vi "Newmark-Home.vi"(0 "Table VRN IN":refnum<visa-resource-name>="COM9", 1 "Comm Active":refnum<vi>, 2 "Exceptions":refnum<vi>, 5 "StageTAGs":string[](array[string]), 7 "Velocities":cluster{"Slow":dbl, "Fast":dbl, "Accel":dbl}={"Slow"=10.0, "Fast"=25000.0, "Accel"=25000.0}, 9 "HomeReverse?":bool[](array[boolean]), 11 "Error IN":errorcluster, 12 "Quit Orgine":refnum<vi>, 13 "EndValues":i32[](array[numeric])) -> (4 "Table VRN OUT":refnum<visa-resource-name>="COM9", 15 "Error OUT":errorcluster)   [LabVIEW 2011]
panel:
  out "NumOT":i32
  out "T Home":dbl
  out "Z Home":dbl
  out "Y Home":dbl
  out "X Home":dbl
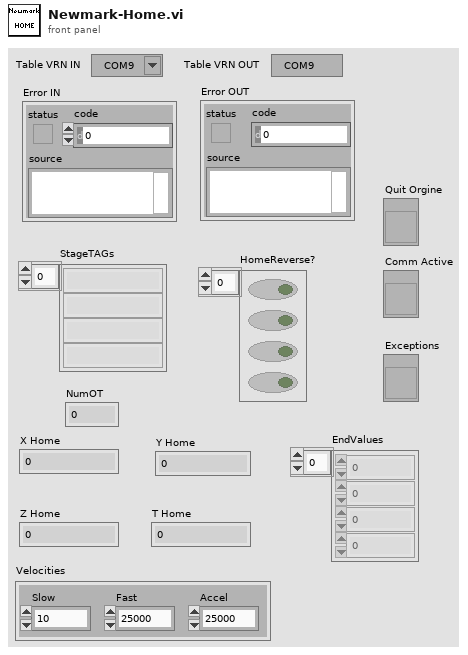
[diagram p1: front panel]
types:
  T1 = cluster{"Command Error":bool, "Slip/Stall":bool, "Overtravel":bool, "Done":bool, "nError":u32, "nSlip":u32, "nOT":u32, "nDone":u32}
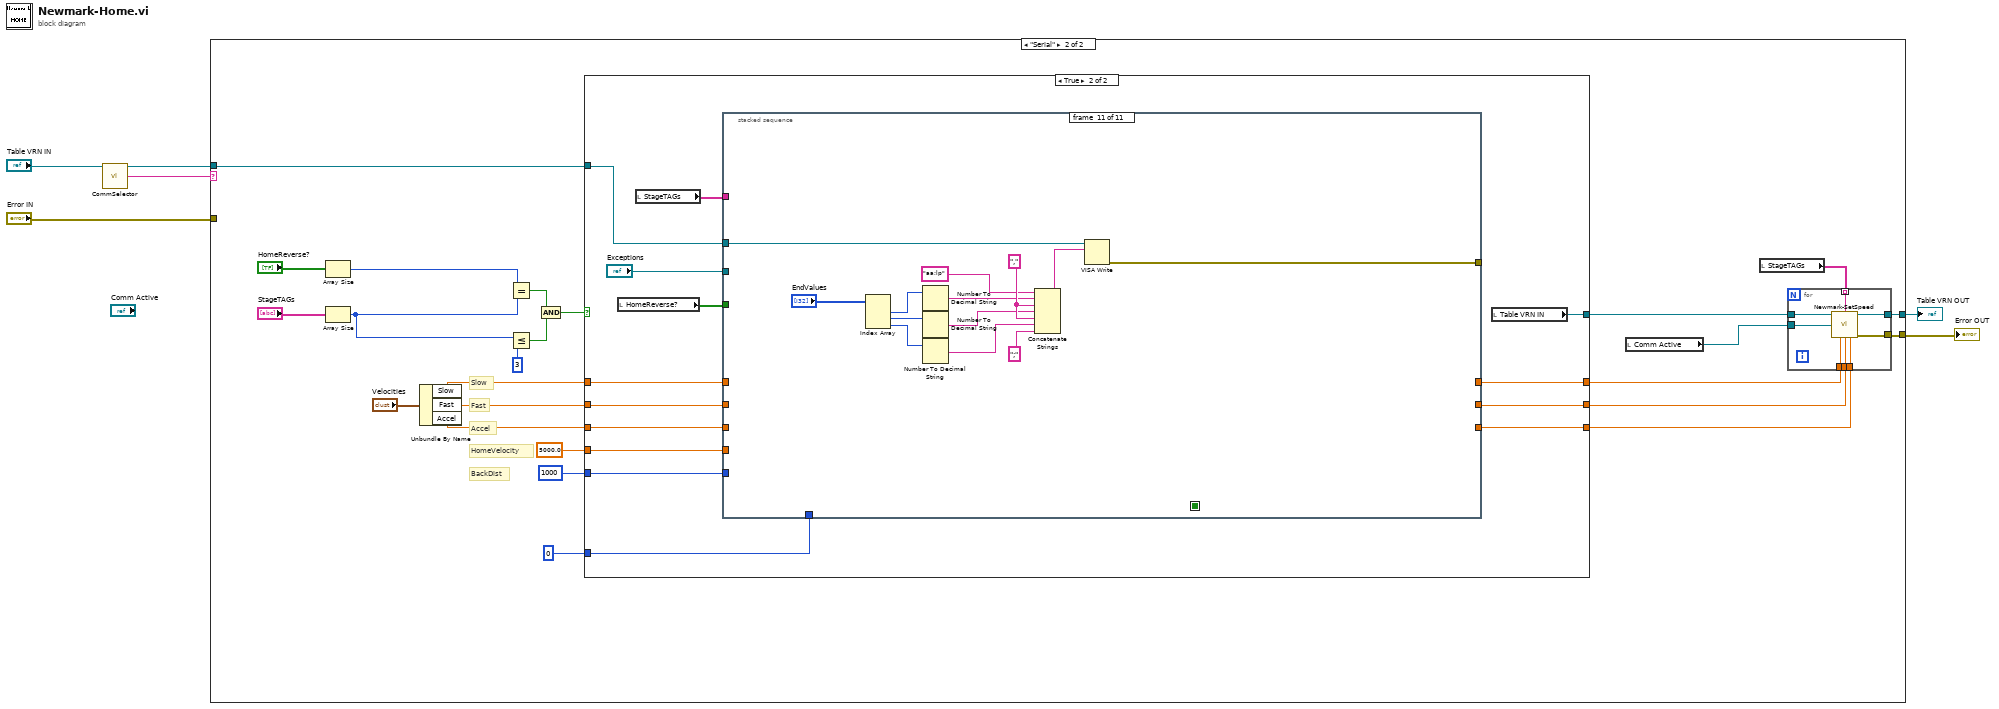
[diagram p0: block diagram]
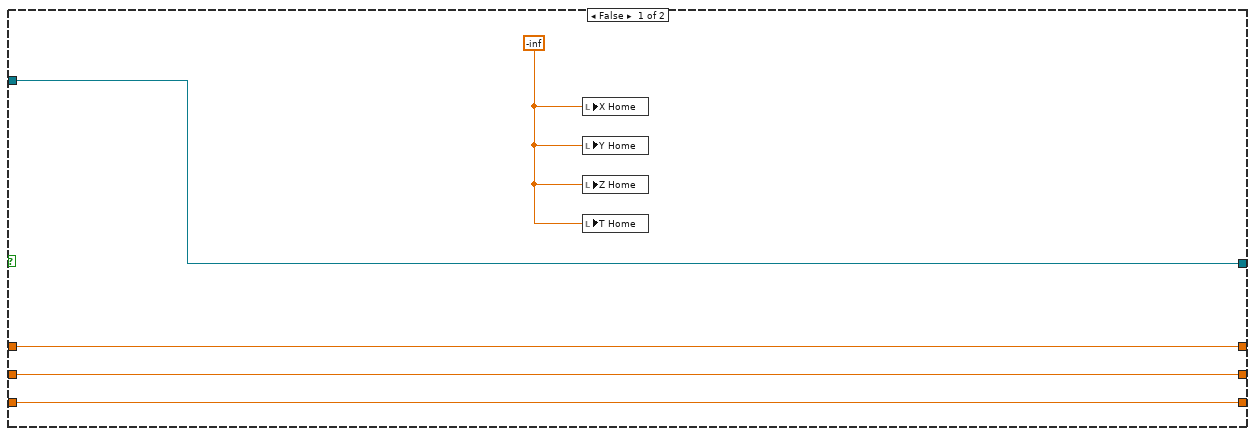
[diagram p3: hidden frame]
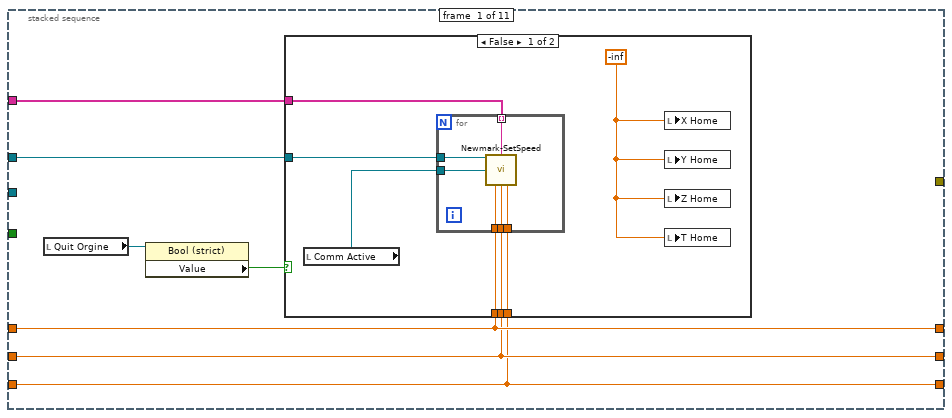
[diagram p4: hidden frame]
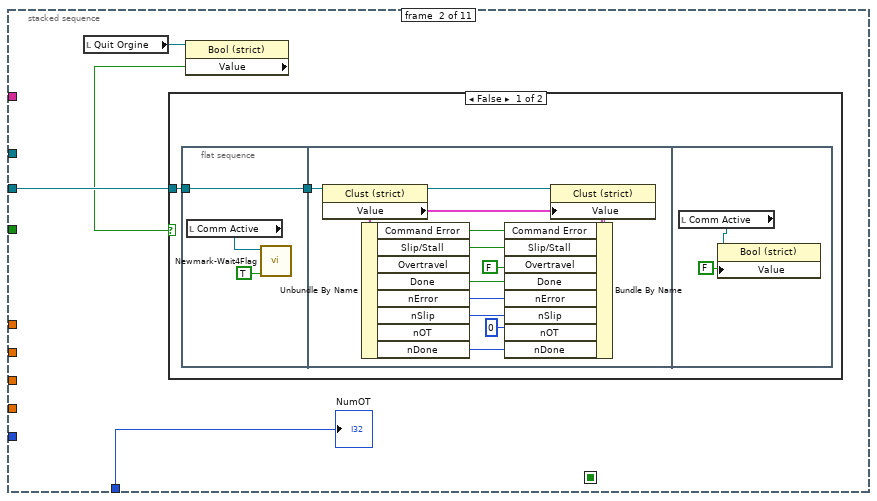
[diagram p6: hidden frame]
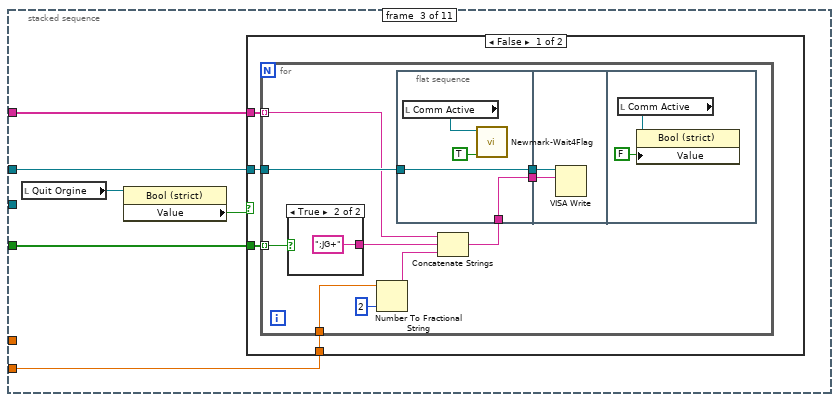
[diagram p8: hidden frame]
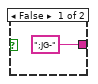
[diagram p9: hidden frame]
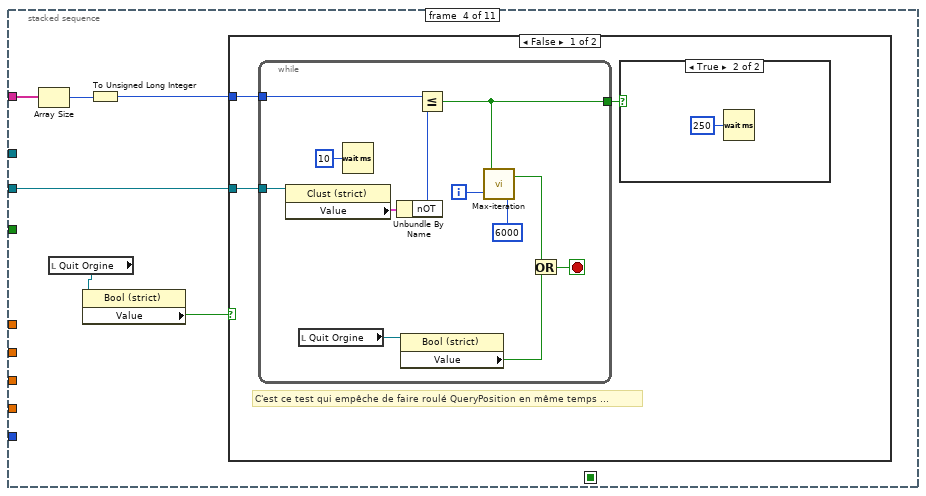
[diagram p11: hidden frame]
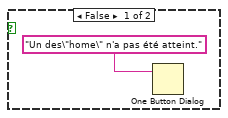
[diagram p12: hidden frame]
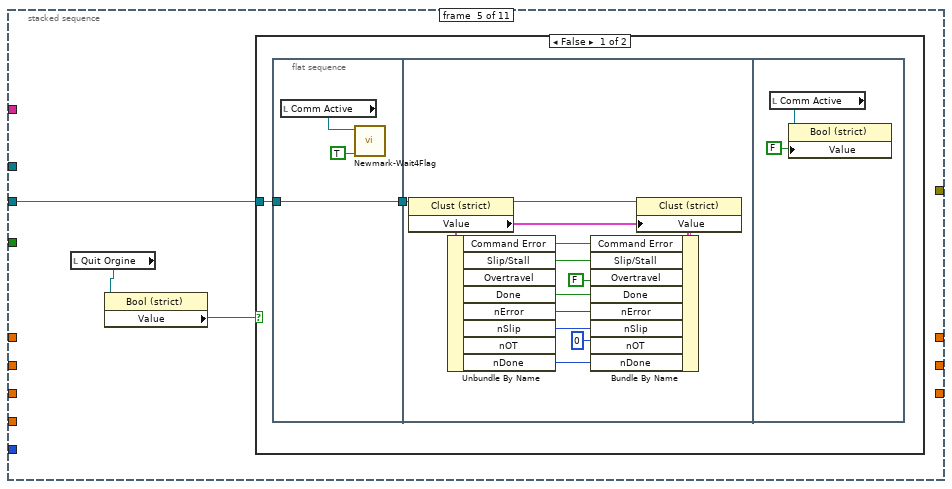
[diagram p14: hidden frame]
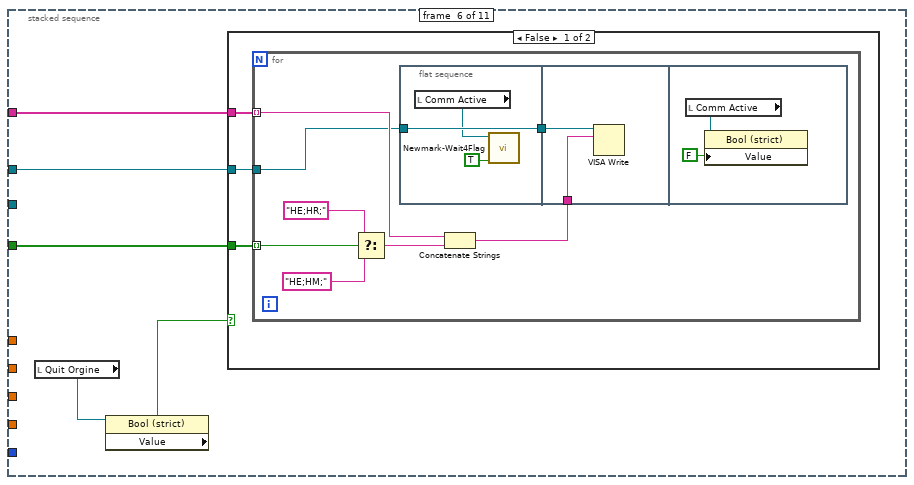
[diagram p16: hidden frame]
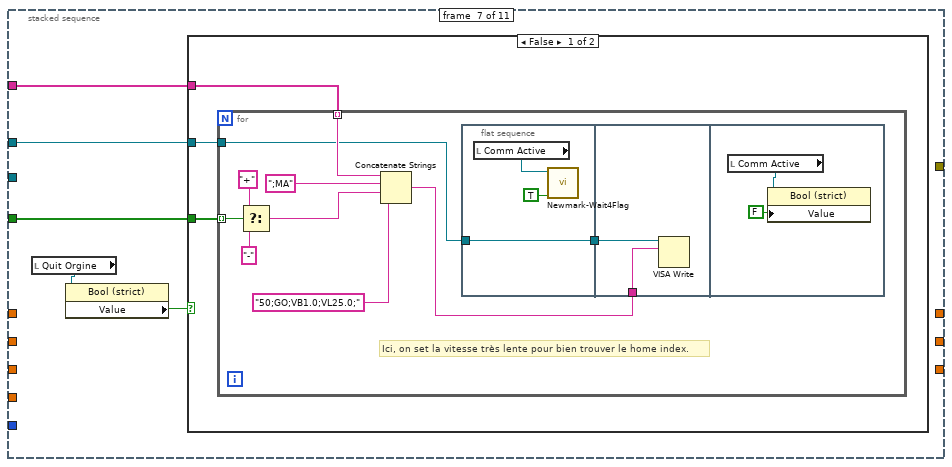
[diagram p18: hidden frame]
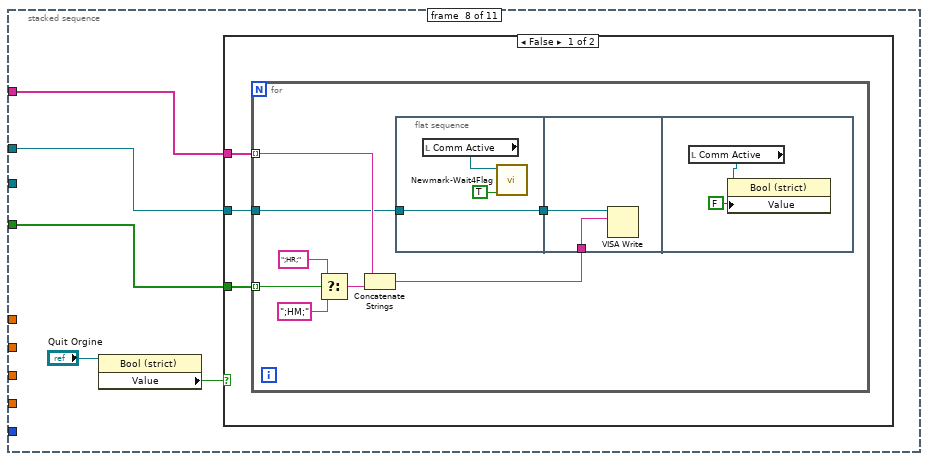
[diagram p20: hidden frame]
diagram:
  n1 = call "CommSelector.vi"("VISA resource name"="Table VRN IN") -> ("VISA resource name"=w3:refnum<visa-resource-name>, "CommType"=w2:string)  [unwired: 13 in]
  n2 = case shown="\"Serial\"" w2 {
    tunnel: w3 -> [w8 w18]
    tunnel: [w8 w16] -> w6
    tunnel: [w7 w11] -> w5
    tunnel: "Error IN" -> [w7 _]
    frame "Unknown", Default {
    }
    frame "Serial" {
      # "Accel"
      # "BackDist"
      # "HomeVelocity"
      # "Fast"
      # "Slow"
      n3 = Array Size(array="HomeReverse?") -> (size(s)=w30:i32)
      n4 = Array Size(array="StageTAGs") -> (size(s)=w23:i32)
      n5 = Unbundle By Name("Velocities") -> ("Slow"=w13:dbl, "Fast"=w14:dbl, "Accel"=w12:dbl)
      n6 = Equal?(x=w30, y=w23) -> (x = y?=w28:bool)
      n7 = Less Or Equal?(x=w23, y=3) -> (x <= y?=w27:bool)
      n8 = And(x=w28, y=w27) -> (x .and. y?=w26:bool)
      n9 = case shown="True" w26 {
        tunnel: w13 -> [w43 w57]
        tunnel: w14 -> [w42 w56]
        tunnel: 5000.0 -> [_ w55]
        tunnel: 1000 -> [_ w54]
        tunnel: w12 -> [w41 w53]
        tunnel: [w43 w52] -> w22
        tunnel: [w42 w51] -> w21
        tunnel: [w41 w50] -> w20
        tunnel: [w44 w49] -> w19
        tunnel: w18 -> [w44 w48]
        tunnel: 0 -> [_ w47]
        frame False {
          w45 = -inf
          n10 = local write "X Home"(w45) -> ()
          n11 = local write "Y Home"(w45) -> ()
          n12 = local write "Z Home"(w45) -> ()
          n13 = local write "T Home"(w45) -> ()
        }
        frame True {
          n14 = local read "HomeReverse?"() -> (w58:bool[])
          n15 = local read "StageTAGs"() -> (w59:string[])
          n16 = stacked-sequence {
            seq-local: [_ _ _ _ _ _ _ _ _ w280 _] -> [_ _ _ _ _ _ _ _ _ _ _]
            tunnel: w59 -> [w66 _ w108 w138 _ w180 w205 w230 _ _ _]
            tunnel: w58 -> [_ _ w107 _ _ w181 w204 w229 _ _ _]
            tunnel: w57 -> [w64 _ _ _ _ _ _ _ _ _ _]
            tunnel: w56 -> [w63 _ w105 _ _ _ _ _ _ _ _]
            tunnel: w55 -> [_ _ _ _ _ _ _ _ _ _ _]
            tunnel: w54 -> [_ _ _ _ _ _ _ _ _ _ _]
            tunnel: w48 -> [w65 _ w106 _ _ w182 w203 w228 w251 w284 w311]
            tunnel: w53 -> [w62 _ _ _ _ _ _ _ _ _ _]
            tunnel: [w64 _ _ _ _ _ _ _ _ _ _] -> w52
            tunnel: [w63 _ _ _ _ _ _ _ _ _ _] -> w51
            tunnel: [w62 _ _ _ _ _ _ _ _ _ _] -> w50
            tunnel: w47 -> [_ w83 _ _ _ _ _ _ _ _ _]
            tunnel: "Exceptions" -> [_ w82 _ w136 w158 _ _ _ _ _ _]
            tunnel: [_ _ _ _ _ _ _ _ _ _ w310] -> _
            frame #0 {
              n17 = local read "Quit Orgine"() -> (w61:refnum<vi>)
              n18 = property class="Bool (strict)"(reference=w61) -> ("Value"=w60:bool)  [unwired: 1 in, 2 out]
              n19 = case shown="False" w60 {
                tunnel: w66 -> [w73 _]
                tunnel: w65 -> [w72 _]
                tunnel: w64 -> [w70 _]
                tunnel: w63 -> [w69 _]
                tunnel: w62 -> [w68 _]
                frame False {
                  w71 = -inf
                  n20 = local read "Comm Active"() -> (w67:refnum<vi>)
                  n21 = for {
                    tunnel: w73 -> [w79] mode=indexing
                    tunnel: w72 -> [w78]
                    tunnel: w70 -> [w77]
                    tunnel: w69 -> [w76]
                    tunnel: w68 -> [w75]
                    tunnel: w67 -> [w74]
                    n22 = call "Newmark-SetSpeed.vi"("Table VRN"=w78, "StageTAG"=w79, "Bool Refnum"=w74, "Vitesse Lente"=w77, "Vitesse Rapide"=w76, "Accélération"=w75) -> ()  [unwired: 7 in, 3 out]
                  }
                  n23 = local write "X Home"(w71) -> ()
                  n24 = local write "Y Home"(w71) -> ()
                  n25 = local write "Z Home"(w71) -> ()
                  n26 = local write "T Home"(w71) -> ()
                }
                frame True {
                }
              }
            }
            frame #1 {
              n27 = local read "Quit Orgine"() -> (w81:refnum<vi>)
              n28 = property class="Bool (strict)"(reference=w81) -> ("Value"=w80:bool)  [unwired: 1 in, 2 out]
              n29 = case shown="False" w80 {
                tunnel: w82 -> [w84 _]
                frame False {
                  n30 = flat-sequence {
                    tunnel: w84 -> [w88]
                    tunnel: [w88] -> w85
                    tunnel: w85 -> [w100]
                    frame #0 {
                      n31 = local read "Comm Active"() -> (w87:refnum<vi>)
                      n32 = call "Newmark-Wait4Flag.vi"("Raise Flag ?"=TRUE, "Ctl Refnum IN"=w87) -> ()  [unwired: 8 in, 2 out]
                    }
                    frame #1 {
                      n33 = property class="Clust (strict)"(reference=w100) -> (reference out=w99:refnum<vi>, "Value"=w98:T1)  [unwired: 1 in, 1 out]
                      n34 = Unbundle By Name(w98) -> ("Command Error"=w96:bool, "Slip/Stall"=w95:bool, "Done"=w92:bool, "nError"=w91:u32, "nSlip"=w90:u32, "nDone"=w89:u32)  [unwired: 2 out]
                      n35 = Bundle By Name(cluster=w98, "Command Error"=w96, "Slip/Stall"=w95, "Overtravel"=FALSE, "Done"=w92, "nError"=w91, "nSlip"=w90, "nOT"=u32 0, "nDone"=w89) -> (w97:T1)
                      n36 = property class="Clust (strict)"(reference=w99, "Value"=w97) -> ()  [unwired: 1 in, 2 out]
                    }
                    frame #2 {
                      n37 = local read "Comm Active"() -> (w102:refnum<vi>)
                      n38 = property class="Bool (strict)"(reference=w102, "Value"=FALSE ("Raise Flag ?")) -> ()  [unwired: 1 in, 2 out]
                    }
                  }
                }
                frame True {
                }
              }
              "NumOT" <- w83
            }
            frame #2 {
              n39 = local read "Quit Orgine"() -> (w104:refnum<vi>)
              n40 = property class="Bool (strict)"(reference=w104) -> ("Value"=w103:bool)  [unwired: 1 in, 2 out]
              n41 = case shown="False" w103 {
                tunnel: w108 -> [w112 _]
                tunnel: w107 -> [w111 _]
                tunnel: w106 -> [w110 _]
                tunnel: w105 -> [w109 _]
                frame False {
                  n42 = for {
                    tunnel: w112 -> [w117] mode=indexing
                    tunnel: w111 -> [w116] mode=indexing
                    tunnel: w110 -> [w122]
                    tunnel: w109 -> [w119]
                    n43 = case shown="True" w116 {
                      tunnel: [";JG-" ";JG+"] -> w115
                      frame False {
                      }
                      frame True {
                      }
                    }
                    n44 = Number To Fractional String(number=w119, precision (6)=i16 2) -> (F-format string=w120:string)  [unwired: 2 in]
                    n45 = flat-sequence {
                      tunnel: w122 -> [w128]
                      tunnel: [w128] -> w118
                      tunnel: [w125] -> w114
                      tunnel: w113 -> [w125]
                      tunnel: w118 -> [w130]
                      tunnel: w114 -> [w129]
                      frame #0 {
                        n46 = local read "Comm Active"() -> (w127:refnum<vi>)
                        n47 = call "Newmark-Wait4Flag.vi"("Raise Flag ?"=TRUE, "Ctl Refnum IN"=w127) -> ()  [unwired: 8 in, 2 out]
                      }
                      frame #1 {
                        n48 = VISA Write(VISA resource name=w130, write buffer=w129) -> ()  [unwired: 1 in, 3 out]
                      }
                      frame #2 {
                        n49 = local read "Comm Active"() -> (w132:refnum<vi>)
                        n50 = property class="Bool (strict)"(reference=w132, "Value"=FALSE) -> ()  [unwired: 1 in, 2 out]
                      }
                    }
                    n51 = Concatenate Strings(w117, w115, w120) -> (w113:string)
                  }
                }
                frame True {
                }
              }
            }
            frame #3 {
              n52 = Array Size(array=w138) -> (size(s)=w137:i32)
              n53 = local read "Quit Orgine"() -> (w134:refnum<vi>)
              n54 = property class="Bool (strict)"(reference=w134) -> ("Value"=w133:bool)  [unwired: 1 in, 2 out]
              n55 = To Unsigned Long Integer(number=w137) -> (unsigned 32bit integer=w135:u32)
              n56 = case shown="False" w133 {
                tunnel: w136 -> [w140 _]
                tunnel: w135 -> [w139 _]
                frame False {
                  # "C'est ce test qui empêche de faire roulé QueryPosition en même temps ..."
                  n57 = while {
                    tunnel: w139 -> [w150]
                    tunnel: [w151] -> w141
                    tunnel: w140 -> [w152]
                    i -> [w154]
                    stop <- w147 stop-if-true
                    n58 = property class="Clust (strict)"(reference=w152) -> ("Value"=w149:T1)  [unwired: 1 in, 2 out]
                    n59 = local read "Quit Orgine"() -> (w145:refnum<vi>)
                    n60 = Wait (ms)(milliseconds to wait=u32 10) -> ()  [unwired: 1 out]
                    n61 = Unbundle By Name(w149) -> ("nOT"=w148:u32)
                    n62 = property class="Bool (strict)"(reference=w145) -> ("Value"=w144:bool)  [unwired: 1 in, 2 out]
                    n63 = Less Or Equal?(x=w150, y=w148) -> (x <= y?=w151:bool)
                    n64 = call "Max-iteration.vi"("i max"=6000, "i act"=w154, "Valeur entrante"=w151) -> ("break ?"=w146:bool)
                    n65 = Or(x=w146, y=w144) -> (x .or. y?=w147:bool)
                  }
                  n66 = case shown="True" w141 {
                    frame False {
                      n67 = One Button Dialog(message="Un des\"home\" n'a pas été atteint.") -> ()  [unwired: 1 in, 1 out]
                    }
                    frame True {
                      n68 = Wait (ms)(milliseconds to wait=u32 250) -> ()  [unwired: 1 out]
                    }
                  }
                }
                frame True {
                }
              }
            }
            frame #4 {
              n69 = local read "Quit Orgine"() -> (w157:refnum<vi>)
              n70 = property class="Bool (strict)"(reference=w157) -> ("Value"=w156:bool)  [unwired: 1 in, 2 out]
              n71 = case shown="False" w156 {
                tunnel: w158 -> [w159 _]
                frame False {
                  n72 = flat-sequence {
                    tunnel: [w161] -> w160
                    tunnel: w159 -> [w161]
                    tunnel: w160 -> [w164]
                    frame #0 {
                      n73 = local read "Comm Active"() -> (w163:refnum<vi>)
                      n74 = call "Newmark-Wait4Flag.vi"("Raise Flag ?"=TRUE, "Ctl Refnum IN"=w163) -> ()  [unwired: 8 in, 2 out]
                    }
                    frame #1 {
                      n75 = property class="Clust (strict)"(reference=w164) -> (reference out=w175:refnum<vi>, "Value"=w174:T1)  [unwired: 1 in, 1 out]
                      n76 = Unbundle By Name(w174) -> ("Command Error"=w172:bool, "Slip/Stall"=w171:bool, "Done"=w168:bool, "nError"=w167:u32, "nSlip"=w166:u32, "nDone"=w165:u32)  [unwired: 2 out]
                      n77 = Bundle By Name(cluster=w174, "Command Error"=w172, "Slip/Stall"=w171, "Overtravel"=FALSE, "Done"=w168, "nError"=w167, "nSlip"=w166, "nOT"=u32 0, "nDone"=w165) -> (w173:T1)
                      n78 = property class="Clust (strict)"(reference=w175, "Value"=w173) -> ()  [unwired: 1 in, 2 out]
                    }
                    frame #2 {
                      n79 = local read "Comm Active"() -> (w177:refnum<vi>)
                      n80 = property class="Bool (strict)"(reference=w177, "Value"=FALSE) -> ()  [unwired: 1 in, 2 out]
                    }
                  }
                }
                frame True {
                }
              }
            }
            frame #5 {
              n81 = local read "Quit Orgine"() -> (w178:refnum<vi>)
              n82 = property class="Bool (strict)"(reference=w178) -> ("Value"=w179:bool)  [unwired: 1 in, 2 out]
              n83 = case shown="False" w179 {
                tunnel: w182 -> [w185 _]
                tunnel: w181 -> [w184 _]
                tunnel: w180 -> [w183 _]
                frame False {
                  n84 = for {
                    tunnel: w185 -> [w188]
                    tunnel: w184 -> [w193] mode=indexing
                    tunnel: w183 -> [w189] mode=indexing
                    n85 = Select(t="HE;HR;", s=w193, f="HE;HM;") -> (s? t:f=w190:string)
                    n86 = flat-sequence {
                      tunnel: w188 -> [w196]
                      tunnel: [w196] -> w186
                      tunnel: w187 -> [w197]
                      tunnel: w186 -> [w198]
                      frame #0 {
                        n87 = local read "Comm Active"() -> (w195:refnum<vi>)
                        n88 = call "Newmark-Wait4Flag.vi"("Raise Flag ?"=TRUE, "Ctl Refnum IN"=w195) -> ()  [unwired: 8 in, 2 out]
                      }
                      frame #1 {
                        n89 = VISA Write(VISA resource name=w198, write buffer=w197) -> ()  [unwired: 1 in, 3 out]
                      }
                      frame #2 {
                        n90 = local read "Comm Active"() -> (w200:refnum<vi>)
                        n91 = property class="Bool (strict)"(reference=w200, "Value"=FALSE) -> ()  [unwired: 1 in, 2 out]
                      }
                    }
                    n92 = Concatenate Strings(w189, w190) -> (w187:string)
                  }
                }
                frame True {
                }
              }
            }
            frame #6 {
              n93 = local read "Quit Orgine"() -> (w202:refnum<vi>)
              n94 = property class="Bool (strict)"(reference=w202) -> ("Value"=w201:bool)  [unwired: 1 in, 2 out]
              n95 = case shown="False" w201 {
                tunnel: w205 -> [w208 _]
                tunnel: w204 -> [w207 _]
                tunnel: w203 -> [w206 _]
                frame False {
                  n96 = for {
                    tunnel: w208 -> [w215] mode=indexing
                    tunnel: w207 -> [w218] mode=indexing
                    tunnel: w206 -> [w209]
                    # "Ici, on set la vitesse très lente pour bien trouver le home index."
                    n97 = Select(t="+", s=w218, f="-") -> (s? t:f=w213:string)
                    n98 = Concatenate Strings(w215, ";MA", w213, "50;GO;VB1.0;VL25.0;") -> (w210:string)
                    n99 = flat-sequence {
                      tunnel: [w219] -> w211
                      tunnel: w209 -> [w219]
                      tunnel: w211 -> [w222]
                      tunnel: w210 -> [w223]
                      frame #0 {
                        n100 = local read "Comm Active"() -> (w221:refnum<vi>)
                        n101 = call "Newmark-Wait4Flag.vi"("Raise Flag ?"=TRUE, "Ctl Refnum IN"=w221) -> ()  [unwired: 8 in, 2 out]
                      }
                      frame #1 {
                        n102 = VISA Write(VISA resource name=w222, write buffer=w223) -> ()  [unwired: 1 in, 3 out]
                      }
                      frame #2 {
                        n103 = local read "Comm Active"() -> (w225:refnum<vi>)
                        n104 = property class="Bool (strict)"(reference=w225, "Value"=FALSE ("Raise Flag ?")) -> ()  [unwired: 1 in, 2 out]
                      }
                    }
                  }
                }
                frame True {
                }
              }
            }
            frame #7 {
              n105 = property class="Bool (strict)"(reference="Quit Orgine") -> ("Value"=w226:bool)  [unwired: 1 in, 2 out]
              n106 = case shown="False" w226 {
                tunnel: w230 -> [w233 _]
                tunnel: w229 -> [w232 _]
                tunnel: w228 -> [w231 _]
                frame False {
                  n107 = for {
                    tunnel: w233 -> [w237] mode=indexing
                    tunnel: w232 -> [w241] mode=indexing
                    tunnel: w231 -> [w235]
                    n108 = Select(t=";HR;", s=w241, f=";HM;") -> (s? t:f=w238:string)
                    n109 = Concatenate Strings(w237, w238) -> (w234:string)
                    n110 = flat-sequence {
                      tunnel: [w242] -> w236
                      tunnel: w235 -> [w242]
                      tunnel: w236 -> [w245]
                      tunnel: w234 -> [w246]
                      frame #0 {
                        n111 = local read "Comm Active"() -> (w244:refnum<vi>)
                        n112 = call "Newmark-Wait4Flag.vi"("Raise Flag ?"=TRUE, "Ctl Refnum IN"=w244) -> ()  [unwired: 8 in, 2 out]
                      }
                      frame #1 {
                        n113 = VISA Write(VISA resource name=w245, write buffer=w246) -> ()  [unwired: 1 in, 3 out]
                      }
                      frame #2 {
                        n114 = local read "Comm Active"() -> (w248:refnum<vi>)
                        n115 = property class="Bool (strict)"(reference=w248, "Value"=FALSE ("Raise Flag ?")) -> ()  [unwired: 1 in, 2 out]
                      }
                    }
                  }
                }
                frame True {
                }
              }
            }
            frame #8 {
              n116 = local read "Quit Orgine"() -> (w250:refnum<vi>)
              n117 = property class="Bool (strict)"(reference=w250) -> ("Value"=w249:bool)  [unwired: 1 in, 2 out]
              n118 = case shown="False" w249 {
                tunnel: w251 -> [w253 _]
                frame False {
                  n119 = local read "Comm Active"() -> (w252:refnum<vi>)
                  n120 = while {
                    tunnel: w253 -> [w278]
                    tunnel: w252 -> [w277]
                    i -> [w259]
                    stop <- w256 stop-if-true
                    n121 = call "Newmark-QueryPosition.vi"("Table VRN IN"=w278, "Bool Refnum"=w277) -> ("X Axis"=w274:dbl, "Y Axis"=w266:dbl, "T Axis"=w261:dbl, "Z Axis"=w264:dbl)  [unwired: 6 in, 4 out]
                    n122 = Absolute Value(x=w274) -> (abs(x)=w276:dbl)
                    n123 = Absolute Value(x=w266) -> (abs(x)=w271:dbl)
                    n124 = Absolute Value(x=w264) -> (abs(x)=w267:dbl)
                    n125 = Absolute Value(x=w261) -> (abs(x)=w270:dbl)
                    n126 = Less Or Equal?(x=w276, y=1.0) -> (x <= y?=w273:bool)
                    n127 = Less Or Equal?(x=w271, y=1.0) -> (x <= y?=w265:bool)
                    n128 = Less Or Equal?(x=w267, y=1.0) -> (x <= y?=w263:bool)
                    n129 = Less Or Equal?(x=w270, y=1.0) -> (x <= y?=w262:bool)
                    n130 = local read "Quit Orgine"() -> (w257:refnum<vi>)
                    n131 = property class="Bool (strict)"(reference=w257) -> ("Value"=w254:bool)  [unwired: 1 in, 2 out]
                    n132 = Compound Arithmetic op=AND(w273, w265, w263, w262) -> (w260:bool)
                    n133 = call "Max-iteration.vi"("i max"=25, "i act"=w259, "Valeur entrante"=w260) -> ("break ?"=w255:bool)
                    n134 = Wait (ms)(milliseconds to wait=u32 200) -> ()  [unwired: 1 out]
                    n135 = Or(x=w255, y=w254) -> (x .or. y?=w256:bool)
                  }
                }
                frame True {
                }
              }
            }
            frame #9 {
              n136 = local read "Quit Orgine"() -> (w283:refnum<vi>)
              n137 = property class="Bool (strict)"(reference=w283) -> ("Value"=w282:bool)  [unwired: 1 in, 2 out]
              n138 = case shown="False" w282 {
                selector: w282 -> [_ w297]
                tunnel: w284 -> [w296 _]
                tunnel: [w285 w297] -> w281
                frame False {
                  w290 = 5.0
                  n139 = local read "Comm Active"() -> (w295:refnum<vi>)
                  n140 = call "Newmark-QueryPosition.vi"("Table VRN IN"=w296, "Bool Refnum"=w295) -> ("X Axis"=w294:dbl, "Y Axis"=w293:dbl, "T Axis"=w291:dbl, "Z Axis"=w292:dbl)  [unwired: 6 in, 4 out]
                  "X Home" <- w294
                  "Y Home" <- w293
                  "T Home" <- w291
                  "Z Home" <- w292
                  n141 = Greater?(x=w294, y=w290) -> (0:w289:bool)
                  n142 = Greater?(x=w293, y=w290) -> (0:w288:bool)
                  n143 = Greater?(x=w292, y=w290) -> (0:w287:bool)
                  n144 = Greater?(x=w291, y=w290) -> (0:w286:bool)
                  n145 = Compound Arithmetic op=OR(w289, w288, w287, w286) -> (w285:bool)
                }
                frame True {
                }
              }
              n146 = Or(x=w281, y=w282) -> (x .or. y?=w280:bool)
              n147 = case shown="False" w280 {
                frame False {
                }
                frame True {
                  n148 = One Button Dialog(message="Problème lors de l'origine des tables ...\n\nVérifier l'état de celles-ci et recommencez.") -> ()  [unwired: 1 in, 1 out]
                }
              }
            }
            frame #10 {
              w308 = "," ("string")
              n149 = Index Array(array="EndValues") -> (element #1=w301:i32, element #2=w302:i32, element #3=w303:i32)  [unwired: 3 in]
              n150 = Number To Decimal String(number=w301) -> (decimal integer string=w304:string)  [unwired: 1 in]
              n151 = Number To Decimal String(number=w302) -> (decimal integer string=w306:string)  [unwired: 1 in]
              n152 = Number To Decimal String(number=w303) -> (decimal integer string=w307:string)  [unwired: 1 in]
              n153 = Concatenate Strings("aa;lp" ("string"), w304, w308, w306, w308, w307, ";" ("string")) -> (w299:string)
              n154 = VISA Write(VISA resource name=w311, write buffer=w299) -> (error out=w310:errorcluster)  [unwired: 1 in, 2 out]
            }
          }
          n155 = local read "Table VRN IN"() -> (w49:refnum<visa-resource-name>)
        }
      }
      n156 = local read "Comm Active"() -> (w10:refnum<vi>)
      n157 = local read "StageTAGs"() -> (w17:string[])
      n158 = for {
        tunnel: w22 -> [w40]
        tunnel: w21 -> [w39]
        tunnel: w20 -> [w38]
        tunnel: w19 -> [w37]
        tunnel: w17 -> [w36] mode=indexing
        tunnel: [w35] -> w16
        tunnel: [w34] -> w11
        tunnel: w10 -> [w33]
        n159 = call "Newmark-SetSpeed.vi"("Table VRN"=w37, "StageTAG"=w36, "Bool Refnum"=w33, "Vitesse Lente"=w40, "Vitesse Rapide"=w39, "Accélération"=w38) -> ("Table VRN OUT"=w35:refnum<visa-resource-name>, "Error OUT"=w34:errorcluster)  [unwired: 7 in, 1 out]
      }
    }
  }
  "Error OUT" <- w5
  "Table VRN OUT" <- w6
